vi "Correlated Digital Output.vi"() -> ()   [LabVIEW 2009]
doc: "I. Description:\nThis example demonstrates how to output a continuous digital pattern using an external clock.\n\nII. Instructions for Running:\n1. Select the Physical Channel to correspond to where your signal is output on the DAQ device.\n2. Select the Clock Source for the generation.\n3. Specify the Rate of the output digital pattern.\n4. Enter the digital pattern data.\n\nIII. Block Diagram Steps:\n1. Create an Digital Output Channel. \n2. Call the DAQmx (Sample Clock) VI which sets the sample clock rate. Additionally, set the sample mode to continuous.\n3. Write the data to the output buffer.\n4. Call the Start VI\n5. Loop continuously until the user presses the Stop button. Check for errors every 100 ms using the Is Task Done? VI\n6. Call the Clear Task VI to clear the Task.\n7. Use the popup dialog box to display an error or warning if any.\n\nIV. I/O Connections Overview:\nMake sure your signal output terminal matches the Physical Channel I/O Control. Also, make sure your external clock terminal matches the Clock Source Control. For further connection information, refer to your hardware reference manual."
uses:
  <vilib>/DAQmx/write.llb/DAQmx Write (Digital 1D U8 1Chan NSamp).vi
  <vilib>/DAQmx/configure/timing.llb/DAQmx Timing (Sample Clock).vi
  <vilib>/DAQmx/create/channels.llb/DAQmx Create Channel (DO-Digital Output).vi
panel:
  in  "lines":tag="Dev1/port0"
  in  "data":u8[](array[numeric])=[1, 2, 4, 8, 16, 32, 64, 128] format="%08b"
  in  "Max AO Clock Rate":dbl=100.0 caption="Sample Clock Rate" format="%.2f"
  in  "AO Sample Clock Source":tag="/Dev1/ao/SampleClock" caption="Clock Source"
  in  "stop":bool
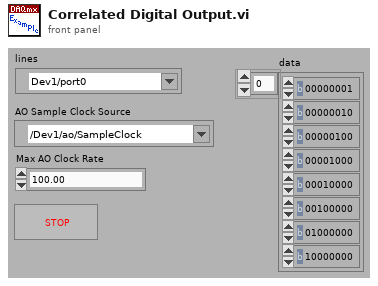
[diagram p1: front panel]
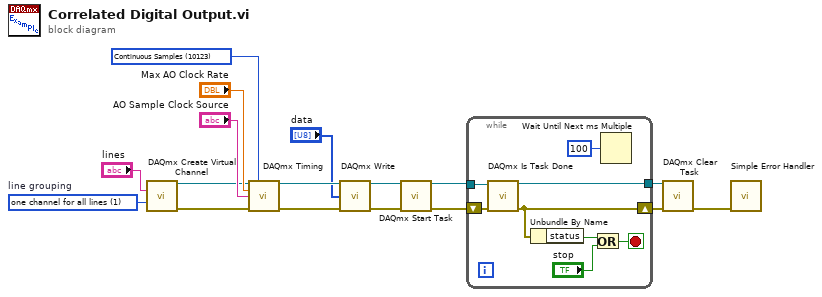
[diagram p0: block diagram]
diagram:
  w6 = 1 items=["one channel for each line", "one channel for all lines"]  # line grouping
  w14 = 10123 items=["Finite Samples"=10178, "Continuous Samples"=10123] ("sample mode")
  n1 = call-poly <vilib>:"DAQmx Create Virtual Channel.vi"("lines"="lines", "line grouping"=w6) -> ("task out"=w4:refnum<k21>, "error out"=w3:errorcluster)  [unwired: 12 in]
  n2 = call-poly <vilib>:"DAQmx Timing.vi"("task/channels in"=w4, "sample mode"=w14, "rate"="Max AO Clock Rate", "source"="AO Sample Clock Source", "error in"=w3) -> ("task out"=w11:refnum<k21>, "error out"=w8:errorcluster)  [unwired: 9 in]
  n3 = call-poly <vilib>:"DAQmx Write.vi"("task/channels in"=w11, "data"="data", "error in"=w8) -> ("task out"=w5:refnum<k21>, "error out"=w13:errorcluster)  [unwired: 10 in, 1 out]
  n4 = call <vilib>:"DAQmx Start Task.vi"("task/channels in"=w5, "error in"=w13) -> ("task out"=w16:refnum<k21>, "error out"=w12:errorcluster)  [unwired: 12 in]
  n5 = while {
    tunnel: w16 -> [w25]
    tunnel: [w24] -> w10
    shift-right: [w21] -> w9
    shift-left: w12 -> [w23]
    stop <- w19 stop-if-true
    n6 = call <vilib>:"DAQmx Is Task Done.vi"("task/channels in"=w25, "error in"=w23) -> ("task out"=w24:refnum<k21>, "error out"=w21:errorcluster)  [unwired: 11 in, 1 out]
    n7 = Unbundle By Name(w21) -> ("status"=w22:bool)
    n8 = Or(x=w22, y="stop") -> (x .or. y?=w19:bool)
    n9 = Wait Until Next ms Multiple(millisecond multiple=u32 100) -> ()  [unwired: 1 out]
  }
  n10 = call <vilib>:"DAQmx Clear Task.vi"("task in"=w10, "error in"=w9) -> ("error out"=w17:errorcluster)  [unwired: 13 in]
  n11 = call <vilib>:"Simple Error Handler.vi"("error in (no error)"=w17) -> ()  [unwired: 4 in, 5 out]
